vi "K 5Baud Init.vi"(6 "pKB2":string, 7 "pKB1":string, 8 "error in (no error)":errorcluster, 9 "Addr":u8, 10 "Channel":u8, 11 "DevHandle":i32) -> (0 "error out":errorcluster, 3 "function return":i32, 4 "pKB2 out":string, 5 "pKB1 out":string)   [LabVIEW 2010, in "usb2k.lvlib"]
doc: "int WINAPI K_5BaudInit(int DevHandle, unsigned char Channel,unsigned char Addr,unsigned char *pKB1,unsigned char *pKB2);"
uses:
  usb2k.lvlib
  examples/Labview/PublicFiles/USB2XXX.dll
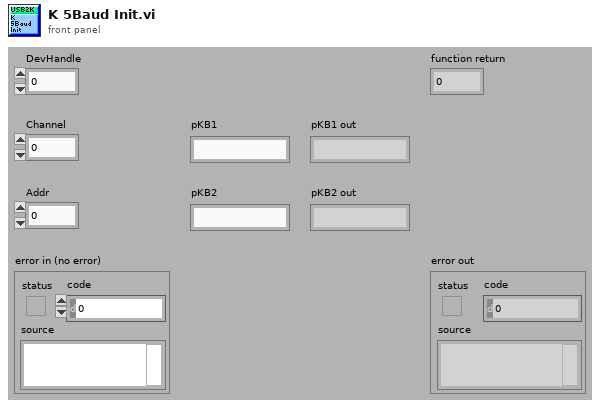
[diagram p1: front panel]
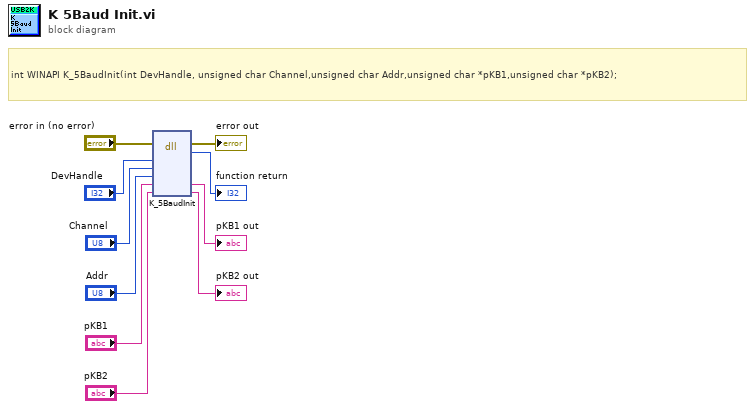
[diagram p0: block diagram]
diagram:
  # "int WINAPI K_5BaudInit(int DevHandle, unsigned char Channel,unsigned char Addr,unsigned char *pKB1,unsigned char *pKB2);"
  n1 = dll-call lib="E:/OtherWork/STM32/USB2XXX_Example/examples/Labview/PublicFiles/USB2XXX.*" fn="K_5BaudInit"(error in="error in (no error)", "DevHandle"="DevHandle", "Channel"="Channel", "Addr"="Addr", "pKB1"="pKB1", "pKB2"="pKB2") -> (error out=→"error out":errorcluster, →"function return":i32, "pKB1"=→"pKB1 out":string, "pKB2"=→"pKB2 out":string)  [unwired: 5 in, 1 out]
